vi "getDofFromFile.vi"(8 "error in (no error)":errorcluster, 10 "DOF Data":path=path "/home/ttsai/Documents/stash/ts_tcs_ofc/testData/sim6_iter1_pert.txt", 11 "OptCtrl in":refnum<class "OptCtrl.lvclass">) -> (0 "error out":errorcluster, 2 "DOF Array":dbl[](array[numeric]), 3 "OptCtrl out":refnum<class "OptCtrl.lvclass">)   [LabVIEW 2016, in "OfcFunc.lvlib" / "OptCtrl.lvclass"]
doc: "Get the degree of freedom (DOF) from file."
uses:
  OptCtrl.lvclass
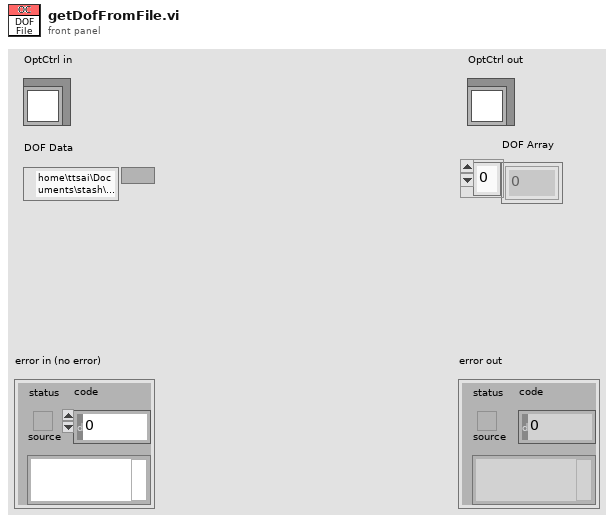
[diagram p1: front panel]
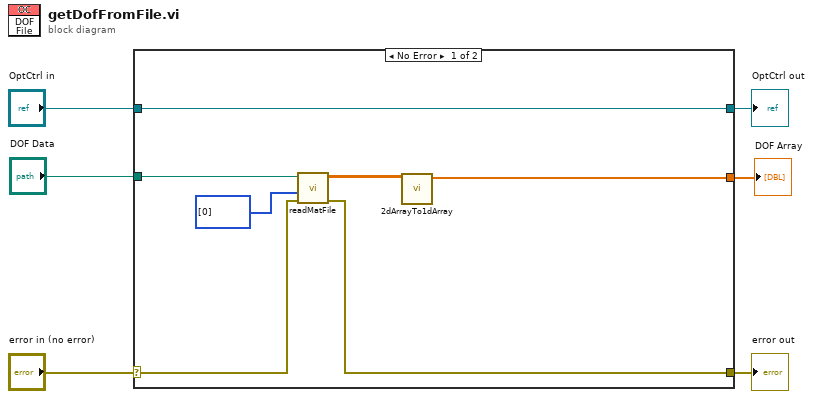
[diagram p0: block diagram]
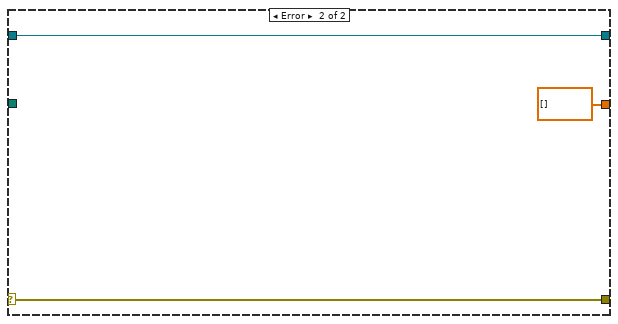
[diagram p2: hidden frame]
diagram:
  n1 = case shown="No Error" "error in (no error)" {
    selector: "error in (no error)" -> [w11 w16]
    tunnel: [w10 w16] -> w5
    tunnel: [w13 w15] -> w3
    tunnel: "OptCtrl in" -> [w13 w15]
    tunnel: "DOF Data" -> [w12 _]
    tunnel: [w9 dbl[] [] ("1D Array")] -> w1
    frame No Error {
      n2 = call "readMatFile.vi"("error in (no error)"=w11, "Skip Col Idx"=i32[] [0], "Path"=w12) -> ("error out"=w10:errorcluster, "Matrix"=w8:dbl[][])  [unwired: 7 in]
      n3 = call "2dArrayTo1dArray.vi"("2D Array"=w8) -> ("1D Array"=w9:dbl[])  [unwired: 10 in]
    }
    frame Error {
    }
  }
  "error out" <- w5
  "OptCtrl out" <- w3
  "DOF Array" <- w1
